vi "piezoWriteOpenNew.vi"() -> ()   [LabVIEW 2017]
uses:
  <vilib>/DAQmx/write.llb/DAQmx Write (Analog DBL 1Chan 1Samp).vi
  <vilib>/DAQmx/write.llb/DAQmx Write (Analog 1D DBL 1Chan NSamp).vi
  globalDevices.vi
  <vilib>/DAQmx/create/channels.llb/DAQmx Create Channel (AO-Voltage-Basic).vi
  <vilib>/DAQmx/configure/timing.llb/DAQmx Timing (Sample Clock).vi
  <vilib>/DAQmx/miscellaneous.llb/DAQmx Fill In Error Info.vi
  Piezo/lvlib/Madlib.lvlib
panel:
  out "function return":i32
  out "Waveform Graph":dbl[](graph)
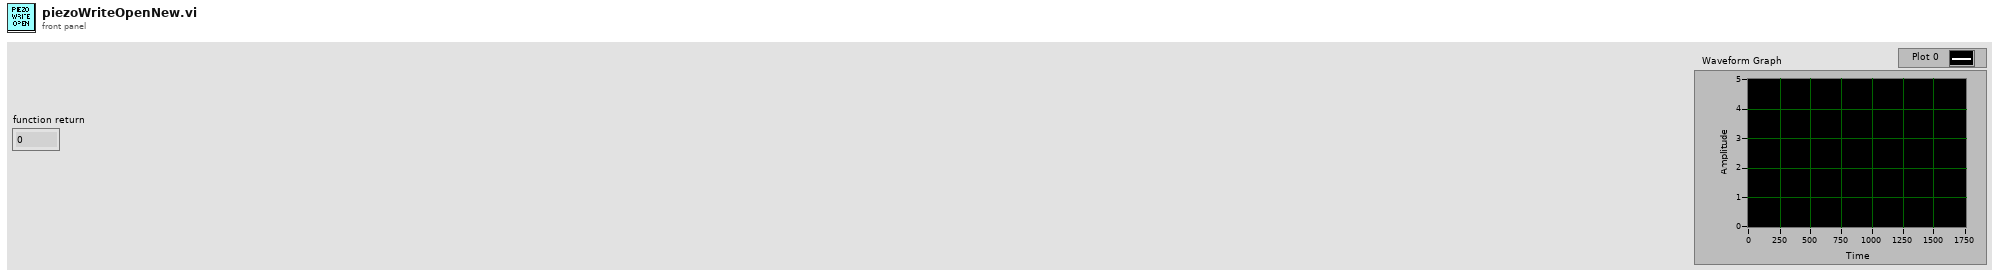
[diagram p1: front panel]
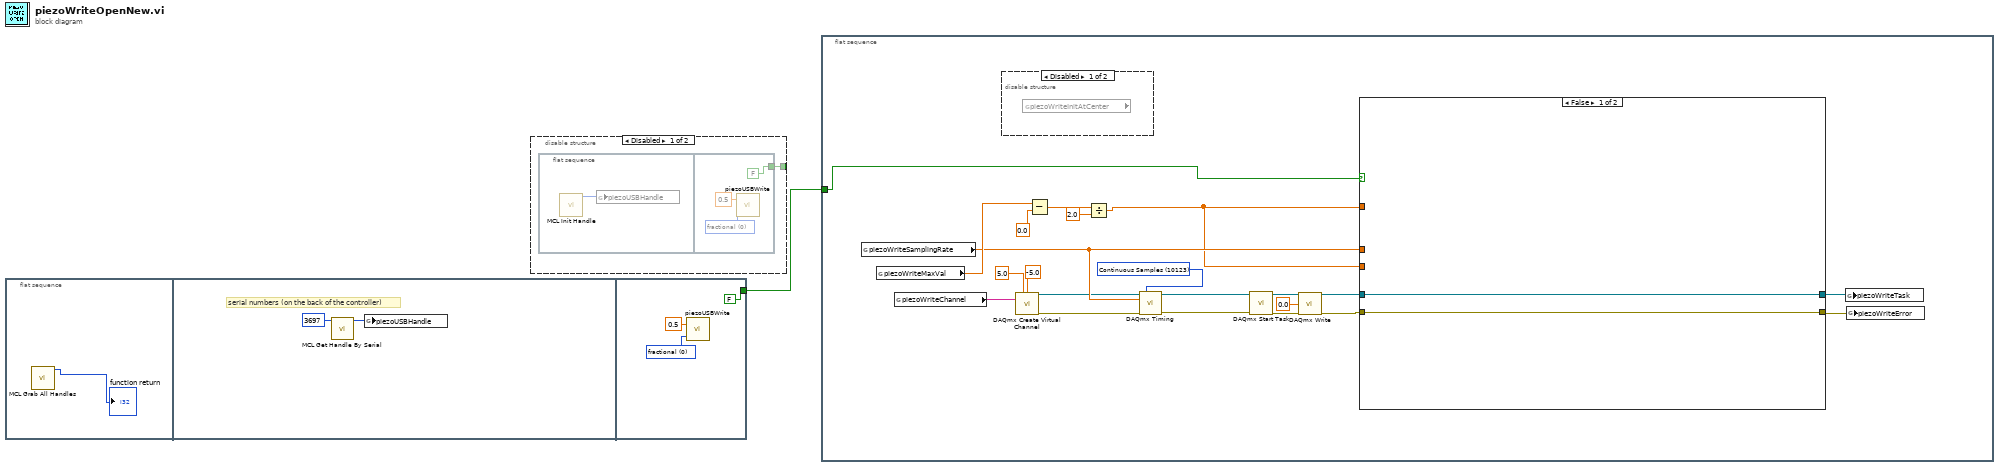
[diagram p0: block diagram]
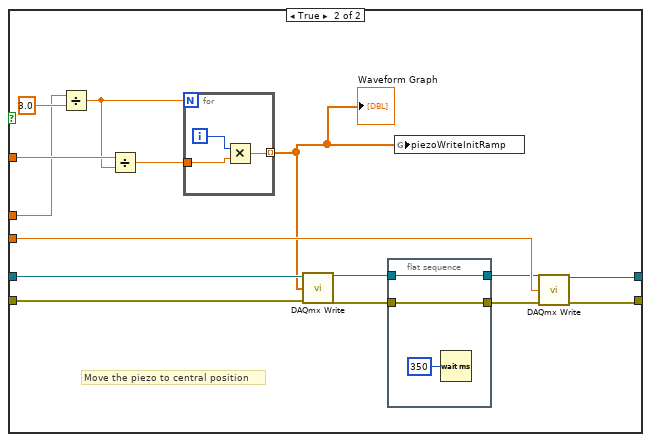
[diagram p4: hidden frame]
diagram:
  n1 = flat-sequence {
    tunnel: [FALSE] -> w1
    frame #0 {
      n2 = call "MCL Grab All Handles.vi"() -> ("function return"=→"function return":i32)  [unwired: 11 in]
    }
    frame #1 {
      # "serial numbers (on the back of the controller)"
      n3 = call "MCL Get Handle By Serial.vi"("serial"=i16 3697) -> ("function return"=w3:i32)  [unwired: 10 in]
      n4 = global write "globalDevices.vi" "piezoUSBHandle"(w3) -> ()
    }
    frame #2 {
      w6 = u16 0 items=["fractional", "voltage (V)", "position (um)"] ("mode")
      n5 = call "piezoUSBWrite.vi"("mode"=w6, "position"=0.5) -> ()  [unwired: 1 in]
    }
  }
  n6 = disable-structure shown="Disabled" {
    disable-tunnel: [w8 _] -> _
    frame Disabled {
      n7 = flat-sequence {
        tunnel: [FALSE] -> w8
        frame #0 {
          n8 = call "MCL Init Handle.vi"() -> ("function return"=w9:i32)  [unwired: 11 in]
          n9 = global write "globalDevices.vi" "piezoUSBHandle"(w9) -> ()
        }
        frame #1 {
          w12 = u16 0 items=["fractional", "voltage (V)", "position (um)"] ("mode")
          n10 = call "piezoUSBWrite.vi"("mode"=w12, "position"=0.5) -> ()  [unwired: 1 in]
        }
      }
    }
    frame Enabled {
    }
  }
  n11 = flat-sequence {
    tunnel: w1 -> [w13]
    frame #0 {
      w27 = 10123 items=["Finite Samples"=10178, "Continuous Samples"=10123, "Hardware Timed Single Point"=12522] ("sample mode")
      n12 = global read "globalDevices.vi" "piezoWriteSamplingRate"() -> (w30:dbl)
      n13 = global read "globalDevices.vi" "piezoWriteMaxVal"() -> (w33:dbl)
      n14 = global read "globalDevices.vi" "piezoWriteChannel"() -> (w34:tag)
      n15 = disable-structure shown="Disabled" {
        frame Disabled {
          n16 = global read "globalDevices.vi" "piezoWriteInitAtCenter"() -> ()  [unwired: 1 out]
        }
        frame Enabled {
        }
      }
      n17 = call-poly <vilib>:"DAQmx Create Virtual Channel.vi"("maximum value"=5.0, "minimum value"=-5.0, "physical channels"=w34) -> ("task out"=w26:refnum<k21>, "error out"=w25:errorcluster)  [unwired: 11 in]
      n18 = Subtract(x=w33, y=0.0 ("minimum value")) -> (x-y=w31:dbl)
      n19 = Divide(x=w31, y=2.0) -> (x/y=w23:dbl)
      n20 = call-poly <vilib>:"DAQmx Timing.vi"("task/channels in"=w26, "sample mode"=w27, "rate"=w30, "error in"=w25) -> ("task out"=w22:refnum<k21>, "error out"=w21:errorcluster)  [unwired: 10 in]
      n21 = call <vilib>:"DAQmx Start Task.vi"("task/channels in"=w22, "error in"=w21) -> ("task out"=w18:refnum<k21>, "error out"=w17:errorcluster)  [unwired: 12 in]
      n22 = call-poly <vilib>:"DAQmx Write.vi"("task/channels in"=w18, "data"=0.0, "error in"=w17) -> ("task out"=w16:refnum<k21>, "error out"=w15:errorcluster)  [unwired: 10 in, 1 out]
      n23 = case shown="False" w13 {
        tunnel: w16 -> [w36 w45]
        tunnel: w15 -> [w35 w46]
        tunnel: w23 -> [_ w50]
        tunnel: w30 -> [_ w47]
        tunnel: [w36 w44] -> w29
        tunnel: [w35 w43] -> w28
        tunnel: w23 -> [_ w42]
        frame False {
        }
        frame True {
          # "Move the piezo to central position"
          n24 = Divide(x=w47, y=3.0) -> (x/y=w49:dbl)
          n25 = Divide(x=w50, y=w49) -> (x/y=w48:dbl)
          n26 = for {
            N: w49 -> [_]
            tunnel: w48 -> [w56]
            tunnel: [w55] -> w37 mode=indexing
            i -> [w57]
            n27 = Multiply(x=w57, y=w56) -> (x*y=w55:dbl)
          }
          "Waveform Graph" <- w37
          n28 = call-poly <vilib>:"DAQmx Write.vi"("task/channels in"=w45, "data"=w37, "error in"=w46) -> ("task out"=w41:refnum<k21>, "error out"=w38:errorcluster)  [unwired: 10 in, 1 out]
          n29 = flat-sequence {
            tunnel: w41 -> [w54]
            tunnel: [w54] -> w40
            tunnel: [w53] -> w39
            tunnel: w38 -> [w53]
            frame #0 {
              n30 = Wait (ms)(milliseconds to wait=u32 350) -> ()  [unwired: 1 out]
            }
          }
          n31 = global write "globalDevices.vi" "piezoWriteInitRamp"(w37) -> ()
          n32 = call-poly <vilib>:"DAQmx Write.vi"("task/channels in"=w40, "data"=w42, "error in"=w39) -> ("task out"=w44:refnum<k21>, "error out"=w43:errorcluster)  [unwired: 10 in, 1 out]
        }
      }
      n33 = global write "globalDevices.vi" "piezoWriteTask"(w29) -> ()
      n34 = global write "globalDevices.vi" "piezoWriteError"(w28) -> ()
    }
  }
